vi "Agilent_Check_Array.vi"(1 "Agilent Array In":T1[](array[typedef])) -> (0 "Any Agilent Bad":bool)   [LabVIEW 2016]
uses:
  AgilentTotalCluster.ctl
  AgilentControl.ctl
  Channel Config.ctl
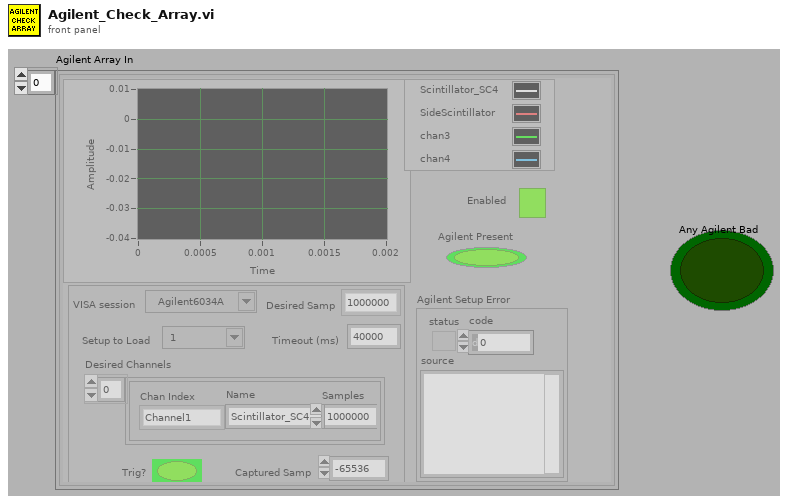
[diagram p1: front panel]
types:
  T1 = typedef "AgilentTotalCluster.ctl" = cluster{"Agilent Graph":waveform(dbl)[], "Agilent Control":T2, "Agilent Setup Error":errorcluster, "Agilent Present":bool, "Enabled":bool}
  T2 = typedef "AgilentControl.ctl" = cluster{"Trig?":bool, "VISA session":refnum<visa-resource-name>, "Setup to Load":string, "Timeout (ms)":u32, "Desired Samp":enum32{"100", "250", "500", "1000", "2000", "5000", "10000", "20000", "50000", "100000", "200000", "500000", "1000000", "2000000", "4000000", "8000000"}, "Captured Samp":i32, "Desired Channels":T3[]}
  T3 = typedef "Channel Config.ctl" = cluster{"Chan Index":enum16{"Channel1", "Channel2", "Channel3", "Channel4", "MATH"}, "Name":string, "Samples":i32}
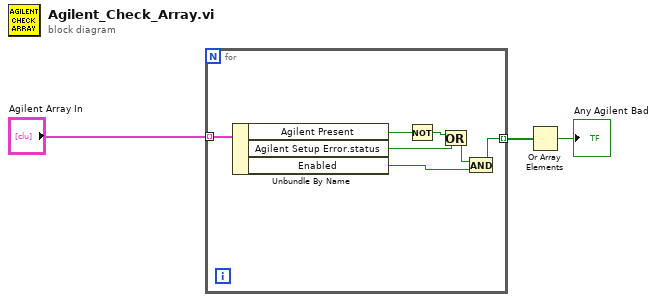
[diagram p0: block diagram]
diagram:
  n1 = for {
    tunnel: "Agilent Array In" -> [w10] mode=indexing
    tunnel: [w4] -> w2 mode=indexing
    n2 = Unbundle By Name(w10) -> ("Agilent Present"=w8:bool, "Agilent Setup Error.status"=w9:bool, "Enabled"=w5:bool)
    n3 = Not(x=w8) -> (.not. x?=w7:bool)
    n4 = Or(x=w7, y=w9) -> (x .or. y?=w6:bool)
    n5 = And(x=w6, y=w5) -> (x .and. y?=w4:bool)
  }
  n6 = Or Array Elements(Boolean array=w2) -> (logical OR=→"Any Agilent Bad":bool)
